vi "vision C.vi"(3 "GIC Input":T1={"     Use ?\nOff       On"=[FALSE, TRUE, FALSE, TRUE], "Mode:"=FALSE, "Extra Port"="", "Hokuyo Port"="COM7", "Tx Prop  Port"="COM6", "Compass Port"="", "GPS Port"="", "Num of WPs"=0, "WP Lats and Longs"={"WP Lats"=[], "WP Longs"=[]}, "Obst Lats and Longs"={"Obst Lats"=[], "Obst Longs"=[]}, "Parameters"=[], "GPS Data"=[], "Compass"=0.0, "LMS Vector"=[], "Vision Vector"=[], "Direction Cmd"=0.0, "Speed Cmd"=0.0, "WP Vector"=[], "WP Number"=0, "Extra"=0, "SW Map"=[], "Path Cluster"={"Path x node"=[], "Path y node"=[]}, "Sim Course"=[]} {"Obst Lats and Longs"."Obst Longs" format="%#_8g"; "Obst Lats and Longs"."Obst Lats" format="%#_8g"}) -> (1 "GIC Output":T1={"     Use ?\nOff       On"=[FALSE, TRUE, FALSE, TRUE], "Mode:"=FALSE, "Extra Port"="", "Hokuyo Port"="COM7", "Tx Prop  Port"="COM6", "Compass Port"="", "GPS Port"="", "Num of WPs"=0, "WP Lats and Longs"={"WP Lats"=[], "WP Longs"=[]}, "Obst Lats and Longs"={"Obst Lats"=[], "Obst Longs"=[]}, "Parameters"=[], "GPS Data"=[], "Compass"=0.0, "LMS Vector"=[], "Vision Vector"=[], "Direction Cmd"=0.0, "Speed Cmd"=0.0, "WP Vector"=[], "WP Number"=0, "Extra"=0, "SW Map"=[], "Path Cluster"={"Path x node"=[], "Path y node"=[]}, "Sim Course"=[]} {"Obst Lats and Longs"."Obst Longs" format="%#_8g"; "Obst Lats and Longs"."Obst Lats" format="%#_8g"})   [LabVIEW 2014]
uses:
  Global_vars.vi
panel:
  out "out":dbl[][](array[numeric])
  in  "Green or Sat Max":dbl(slide)=84.70890410958904 scale=0.0..255.0
  in  "Blue or Luma Max":dbl(slide)=224.43493150684932 scale=0.0..255.0
  in  "Red or Hue Max":dbl(slide)=255.0 scale=0.0..255.0
  in  "Green or Sat Min":dbl(slide) scale=0.0..255.0
  in  "Blue or Luma Min":dbl(slide)=53.27054794520548 scale=0.0..255.0
  in  "Red or Hue Min":dbl(slide)=99.55479452054794 scale=0.0..255.0
  out "image out 2":T2(plugin-control)
  out "loop time":dbl=48.0
  in  "Stop (F)":bool
  out "image out":T2(plugin-control)
  # "Input:"
  # "Output:"
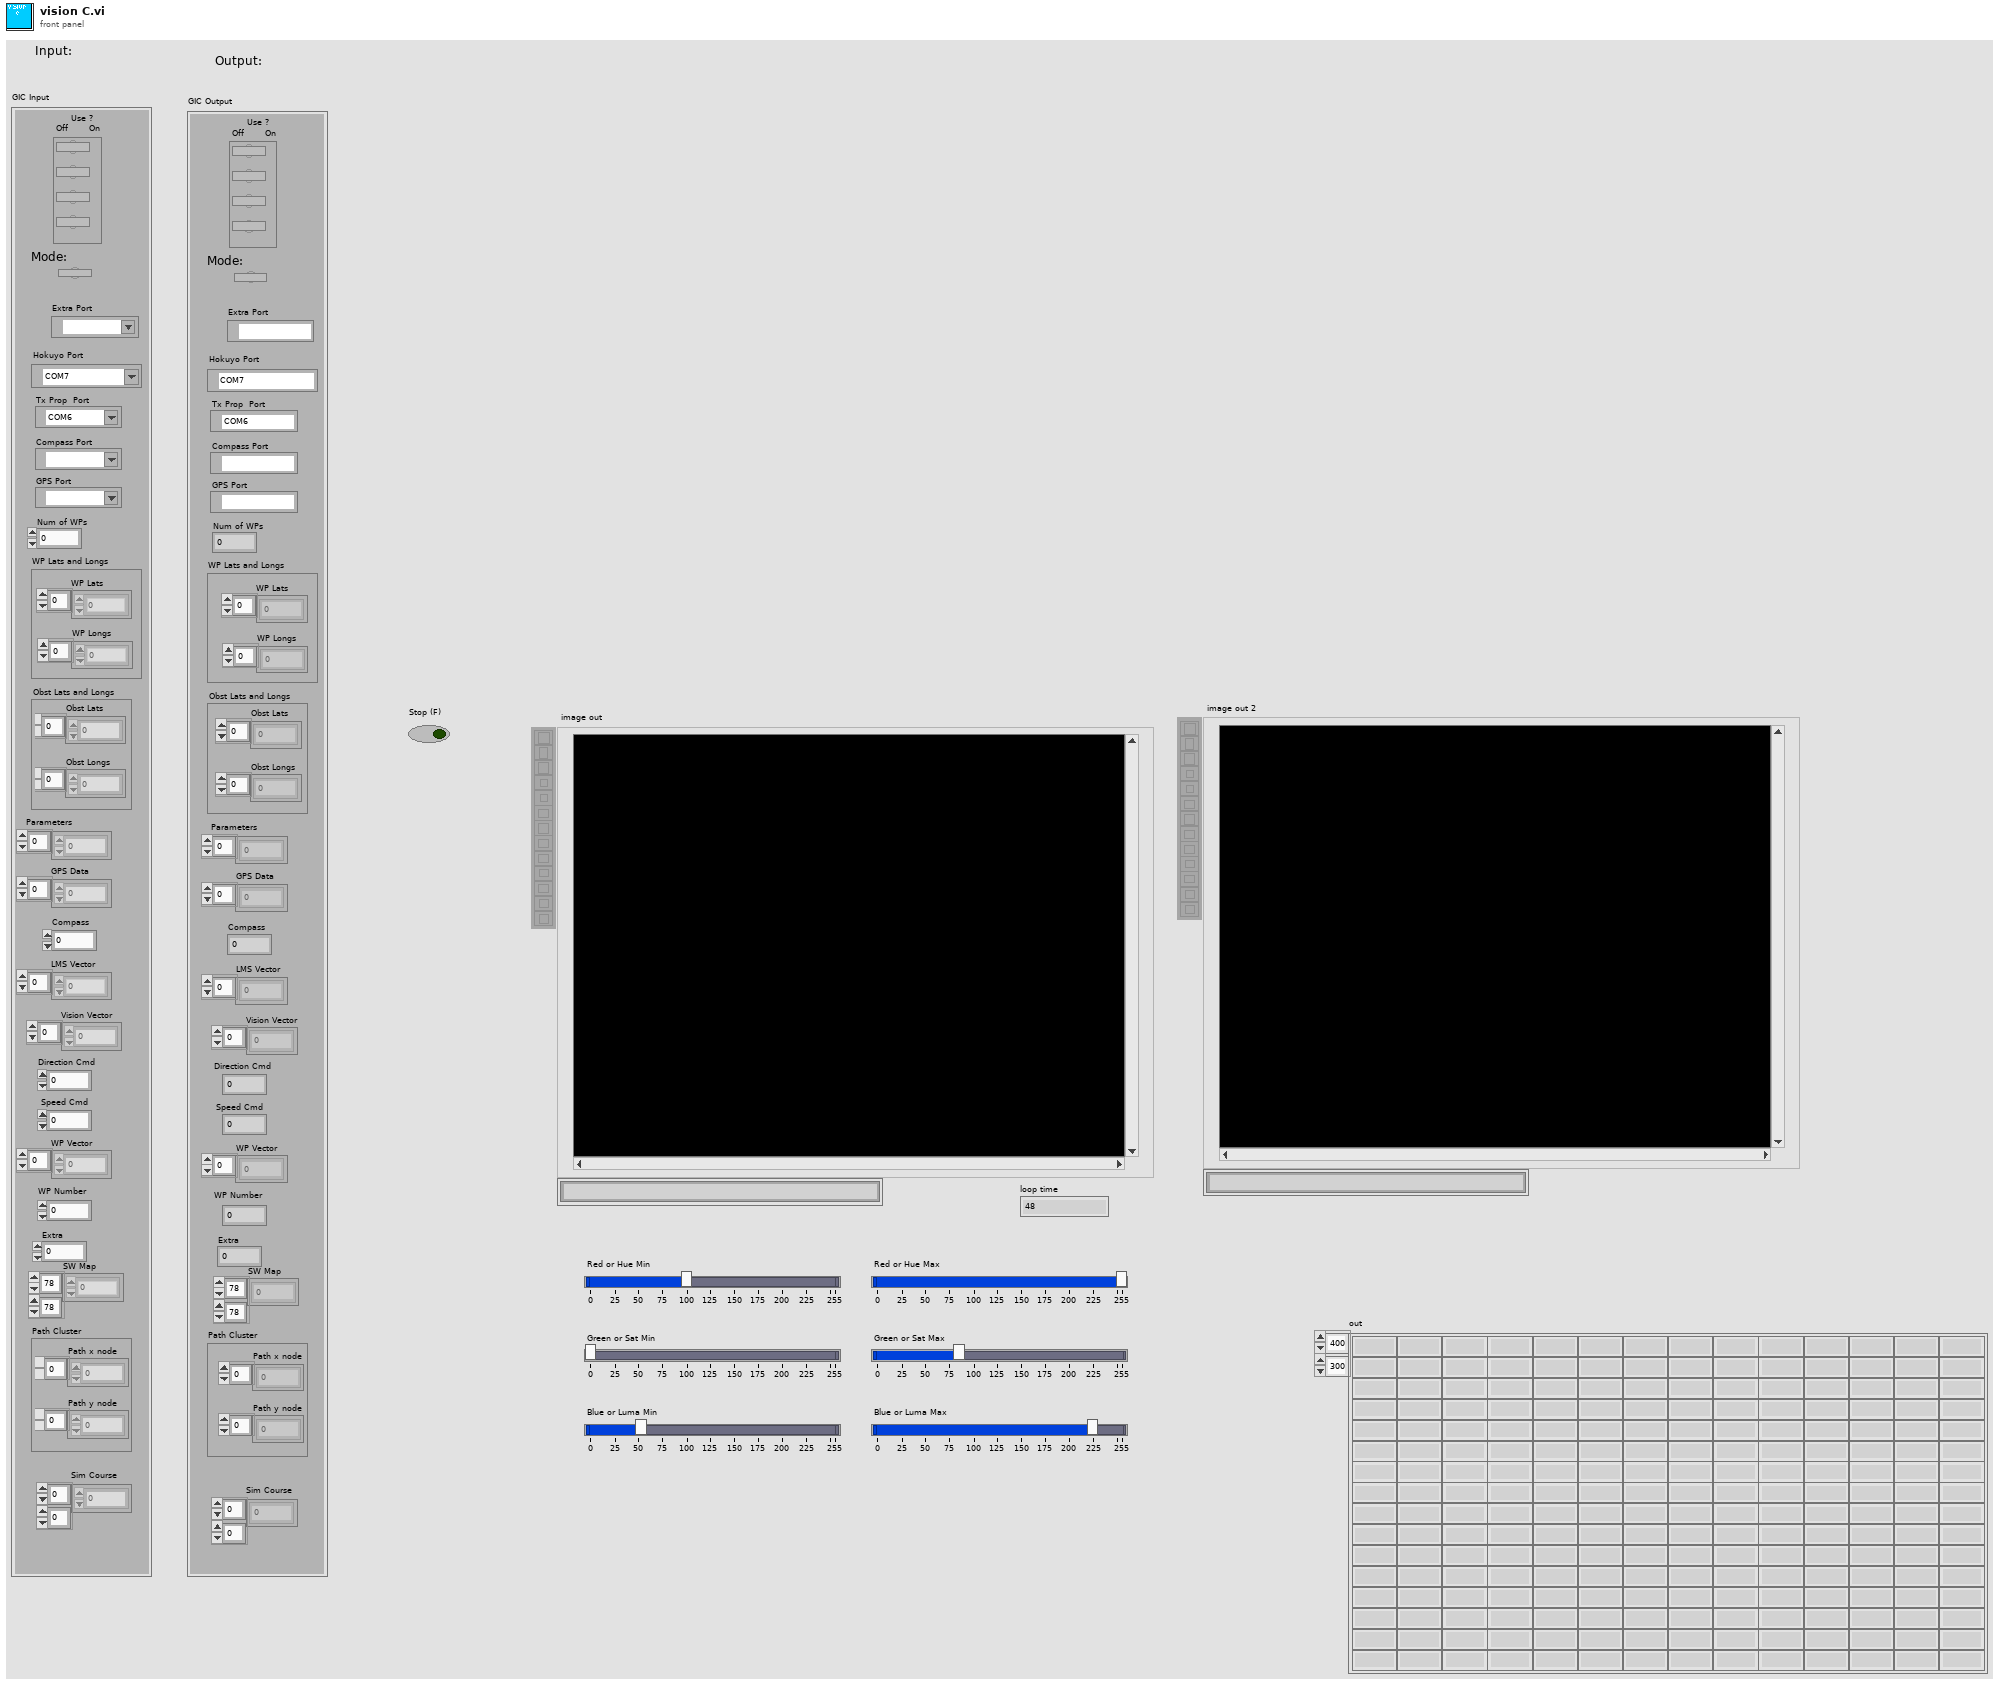
[diagram p1: front panel]
types:
  T1 = cluster{"     Use ?\nOff       On":bool[], "Mode:":bool, "Extra Port":refnum<visa-resource-name>, "Hokuyo Port":refnum<visa-resource-name>, "Tx Prop  Port":refnum<visa-resource-name>, "Compass Port":refnum<visa-resource-name>, "GPS Port":refnum<visa-resource-name>, "Num of WPs":i16, "WP Lats and Longs":cluster{"WP Lats":dbl[], "WP Longs":dbl[]}, "Obst Lats and Longs":cluster{"Obst Lats":dbl[], "Obst Longs":dbl[]}, "Parameters":dbl[], "GPS Data":dbl[], "Compass":dbl, "LMS Vector":dbl[], "Vision Vector":dbl[], "Direction Cmd":dbl, "Speed Cmd":dbl, "WP Vector":dbl[], "WP Number":i32, "Extra":i16, "SW Map":i32[][], "Path Cluster":cluster{"Path x node":dbl[], "Path y node":dbl[]}, "Sim Course":i8[][]}
  T2 = typedef "IMAQ Image.ctl" = refnum<image>
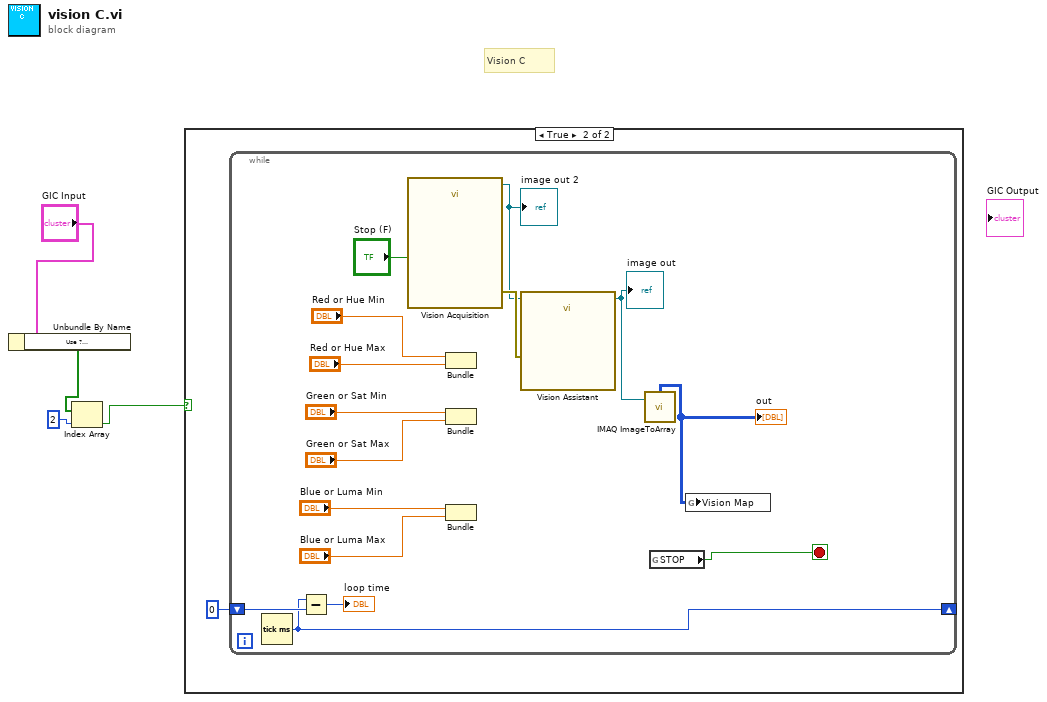
[diagram p0: block diagram]
diagram:
  # "Vision C"
  n1 = Unbundle By Name("GIC Input") -> ("Use ?\nOff       On"=w3:bool[])
  n2 = Index Array(array=w3, index=2) -> (element=w1:bool)
  n3 = case shown="True" w1 {
    frame False {
    }
    frame True {
      n4 = while {
        shift-right: [w16] -> _
        shift-left: 0 -> [w18]
        stop <- w6 stop-if-true
        n5 = Tick Count (ms)() -> (millisecond timer value=w16:u32)
        n6 = Subtract(x=w16, y=w18) -> (x-y=→"loop time":u32)
        n7 = call "Vision Acquisition"("Stop (F)"="Stop (F)") -> ("Image Out"=w15:T2, "error out"=w19:errorcluster)  [unwired: 24 in, 1 out]
        "image out 2" <- w15
        n8 = Bundle("Red or Hue Min"="Red or Hue Min", "Red or Hue Max"="Red or Hue Max") -> ()  [unwired: 1 in, 1 out]
        n9 = Bundle("Green or Sat Min"="Green or Sat Min", "Green or Sat Max"="Green or Sat Max") -> ()  [unwired: 1 in, 1 out]
        n10 = Bundle("Blue or Luma Min"="Blue or Luma Min", "Blue or Luma Max"="Blue or Luma Max") -> ()  [unwired: 1 in, 1 out]
        n11 = call "Vision Assistant"("Image In"=w15, "error in"=w19) -> ("Image Out"=w8:T2)  [unwired: 24 in, 1 out]
        "image out" <- w8
        n12 = call "IMAQ ImageToArray"("Image"=w8) -> ("Image Pixels (U8)"=w7:u8[][])  [unwired: 3 in, 4 out]
        "out" <- w7
        n13 = global read "Global_vars.vi" "STOP"() -> (w6:bool)
        n14 = global write "Global_vars.vi" "Vision Map"(w7) -> ()
      }
    }
  }
